vi "Serrure_Var.vi"() -> ()   [LabVIEW 2018]
panel:
  in  "String":string
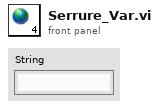
[diagram p1: front panel]
diagram:
